vi "Test_Status_Update.vi"(10 "GKÇ-1 Test Status":T1={"Return Code"=0, "Message"="", "error in (no error)"={"status"=FALSE, "code"=0, "source"=""}, "Program State"=enum."Ön Yükleme Tamam", "Test A. Suresi"=0}) -> (0 "error out":errorcluster)   [LabVIEW 2014]
uses:
  CustomControls/TSE_Status.ctl
  CustomControls/Program_States.ctl
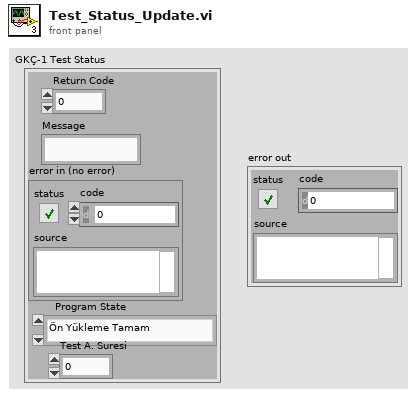
[diagram p1: front panel]
types:
  T1 = typedef "TSE_Status.ctl" = cluster{"Return Code":i32, "Message":string, "error in (no error)":errorcluster, "Program State":T2, "Test A. Suresi":u32}
  T2 = typedef "Program_States.ctl" = enum16{"Ön Yükleme", "TSE Baslat", "Kalibratöre Baglan", "Kalibratörü Baslat", "Ön Yükleme Tamam", "Frekans Testi", "Gerilim Testi", "Akim Testi", "Aktif Guc Testi", "Reaktif Guc Testi", "AC Akim Harmonik Testi", "AC Gerilim Harmonik Testi", "Flicker Testi", "Rapor Cikarma", "Yeniden Başlat", "Bekleme", "Durdur"}
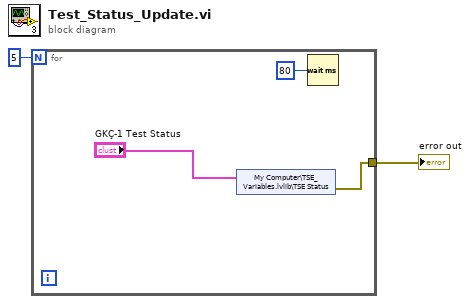
[diagram p0: block diagram]
diagram:
  n1 = for {
    N: 5 -> [_]
    tunnel: [w3] -> w1
    n2 = shared-variable "My Computer\\TSE_Variables.lvlib\\TSE Status"("GKÇ-1 Test Status") -> (error out=w3:errorcluster)  [unwired: 1 in]
    n3 = Wait (ms)(milliseconds to wait=u32 80) -> ()  [unwired: 1 out]
  }
  "error out" <- w1
